vi "Write Logout.vi"(8 "error in (no error)":errorcluster, 10 "Logout":refnum<vi>, 11 "View Manager in":refnum<class "View Manager.lvclass">) -> (0 "error out":errorcluster, 3 "View Manager out":refnum<class "View Manager.lvclass">)   [LabVIEW 2017, in "View Manager.lvlib" / "View Manager.lvclass"]
uses:
  <vilib>/gpm_packages/@cs/User Manager App/View Manager/View Manager/View Manager.lvclass
  <vilib>/gpm_packages/@cs/User Manager App/View Manager/View Manager/View Manager.lvclass/View Manager.ctl
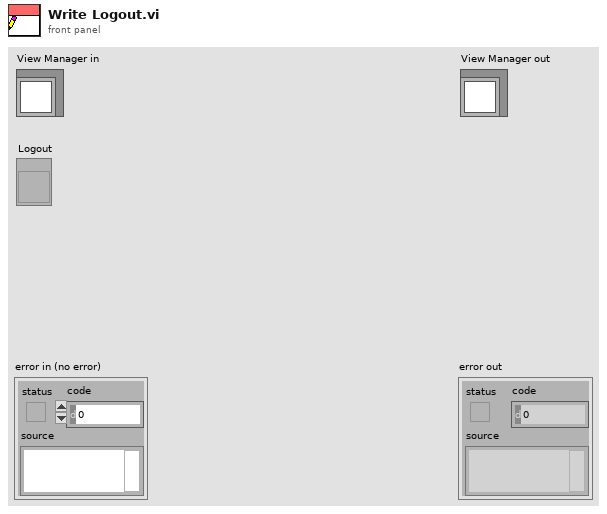
[diagram p1: front panel]
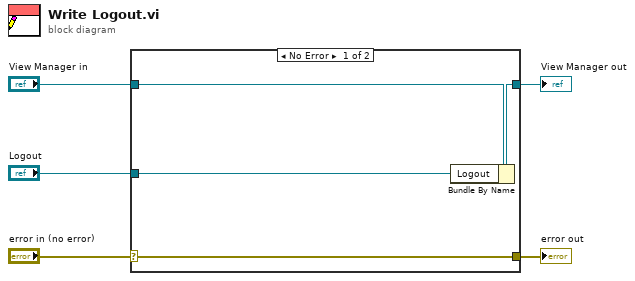
[diagram p0: block diagram]
diagram:
  n1 = case shown="No Error" "error in (no error)" {
    selector: "error in (no error)" -> [w9 w10]
    tunnel: [w9 w10] -> w4
    tunnel: [w7 w11] -> w2
    tunnel: "View Manager in" -> [w8 w11]
    tunnel: "Logout" -> [w6 _]
    frame No Error {
      n2 = Bundle By Name(cluster=w8, "Logout"=w6) -> (w7:refnum<class "View Manager.lvclass">)
    }
    frame Error {
    }
  }
  "error out" <- w4
  "View Manager out" <- w2
